vi "RWSkylinePrefCluster.vi"(7 "Task":enum16{"Read", "Write"}(ring), 8 "error in (no error)":errorcluster, 11 "Device In":T1={"Name"="", "BaseURL"="", "AppKey"="", "Headers"=["Content-Type:application/json"], "Timeout"=10000}) -> (0 "error out":errorcluster, 3 "Device Out":T1={"Name"="", "BaseURL"="", "AppKey"="", "Headers"=["Content-Type:application/json"], "Timeout"=10000})   [LabVIEW 2016]
uses:
  SkylineCluster.ctl
panel:
  out "text":string
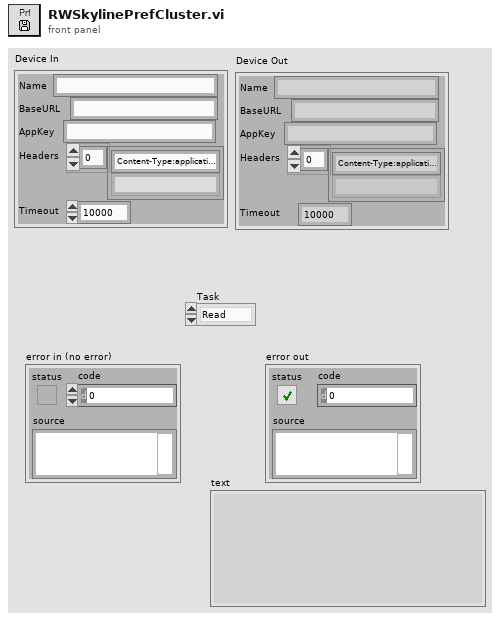
[diagram p1: front panel]
types:
  T1 = typedef "SkylineCluster.ctl" = cluster{"Name":string, "BaseURL":string, "AppKey":string, "Headers":string[], "Timeout":i32}
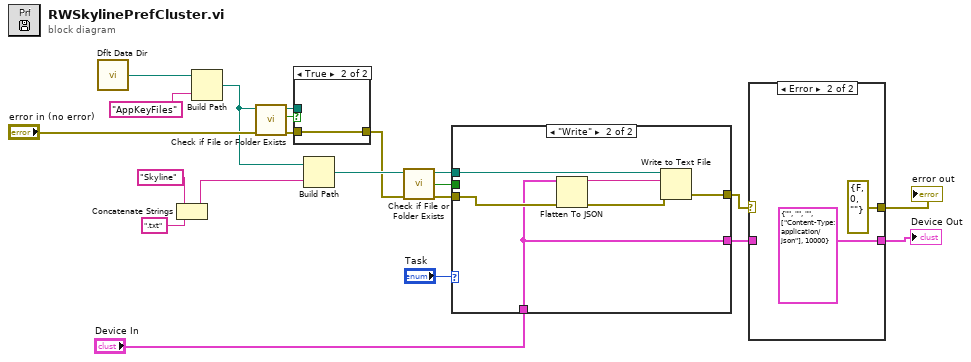
[diagram p0: block diagram]
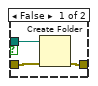
[diagram p2: hidden frame]
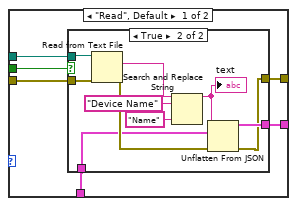
[diagram p4: hidden frame]
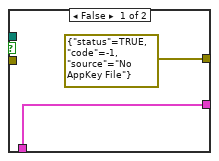
[diagram p5: hidden frame]
diagram:
  n1 = call <vilib>:"Dflt Data Dir.vi"() -> ("App:Default Data Directory"=w6:path)
  n2 = Concatenate Strings("Skyline" ("Name"), ".txt" ("string")) -> (w20:string)
  n3 = Build Path(base path=w6, name or relative path="AppKeyFiles") -> (appended path=w2:path)
  n4 = call <vilib>:"Check if File or Folder Exists.vi"("error in (no error)"="error in (no error)", "path"=w2) -> ("error out"=w3:errorcluster, "file or folder exists?"=w5:bool, "dup path"=w4:path)  [unwired: 7 in]
  n5 = case shown="True" w5 {
    tunnel: w4 -> [w24 _]
    tunnel: w3 -> [w23 w25]
    tunnel: [w22 w25] -> w12
    frame False {
      n6 = Create Folder(path (use dialog)=w24, error in=w23) -> (error out=w22:errorcluster)  [unwired: 1 in, 2 out]
    }
    frame True {
    }
  }
  n7 = Build Path(base path=w2, name or relative path=w20) -> (appended path=w19:path)
  n8 = call <vilib>:"Check if File or Folder Exists.vi"("error in (no error)"=w12, "path"=w19) -> ("error out"=w17:errorcluster, "file or folder exists?"=w15:bool, "dup path"=w18:path)  [unwired: 7 in]
  n9 = case shown="\"Write\"" "Task" {
    tunnel: w18 -> [w30 w49]
    tunnel: w17 -> [w31 w47]
    tunnel: [w29 w45] -> w11
    tunnel: w15 -> [w28 _]
    tunnel: [w27 w44] -> w9
    tunnel: "Device In" -> [w26 w44]
    frame "Read", Default {
      n10 = case shown="True" w28 {
        tunnel: w31 -> [_ w43]
        tunnel: w30 -> [_ w42]
        tunnel: [errorcluster {"status"=TRUE, "code"=-1, "source"="No AppKey File"} ("error out") w38] -> w29
        tunnel: [w32 w39] -> w27
        tunnel: w26 -> [w32 w40]
        frame False {
        }
        frame True {
          n11 = Read from Text File(file (use dialog)=w42, error in=w43) -> (text=w37:string, error out=w41:errorcluster)  [unwired: 2 in, 2 out]
          n12 = Search and Replace String(input string=w37, search string="Device Name", replace string="Name" ("replace string (\"\")")) -> (result string=w34:string)  [unwired: 5 in, 3 out]
          "text" <- w34
          n13 = Unflatten From JSON(JSON string=w34, type and defaults=w40, error in (no error)=w41) -> (value=w39:T1, error out=w38:errorcluster)  [unwired: 4 in]
        }
      }
    }
    frame "Write" {
      n14 = Flatten To JSON(anything=w44, error in (no error)=w47) -> (JSON string=w48:string, 11:w46:errorcluster)  [unwired: 1 in]
      n15 = Write to Text File(file (use dialog)=w49, text=w48, error in=w46) -> (error out=w45:errorcluster)  [unwired: 1 in, 2 out]
    }
  }
  n16 = case shown="Error" w11 {
    selector: w11 -> [w50 _]
    tunnel: [w51 T1 {"Name"="", "BaseURL"="", "AppKey"="", "Headers"=["Content-Type:application/json"], "Timeout"=10000} ("Device In")] -> w10
    tunnel: w9 -> [w51 _]
    tunnel: [w50 errorcluster {"status"=FALSE, "code"=0, "source"=""} ("error IO")] -> w8
    frame No Error {
    }
    frame Error {
    }
  }
  "error out" <- w8
  "Device Out" <- w10
